vi "MW100 General Start.vi"(8 "error in (no error)":errorcluster, 11 "MW100 Input":refnum<visa-resource-name>) -> (0 "error out":errorcluster, 3 "MW100 Output":refnum<visa-resource-name>="MW100")   [LabVIEW 2016]
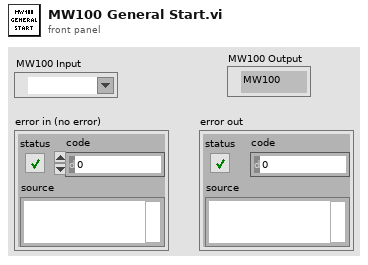
[diagram p1: front panel]
types:
  T1 = enum16{"Computation Start", "Computation stop", "Reset Computation", "Clear Computation"}
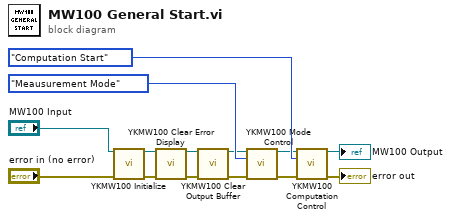
[diagram p0: block diagram]
diagram:
  n1 = call "YKMW100 Initialize.vi"("VISA session (TCPIP::)"="MW100 Input", "error in (no error)"="error in (no error)") -> ("dup VISA session"=w11:refnum<visa-resource-name>, "error out"=w8:errorcluster)  [unwired: 12 in]
  n2 = call "YKMW100 Clear Error Display.vi"("VISA session"=w11, "error in (no error)"=w8) -> ("dup VISA session"=w10:refnum<visa-resource-name>, "error out"=w9:errorcluster)  [unwired: 10 in, 2 out]
  n3 = call "YKMW100 Clear Output Buffer.vi"("VISA session"=w10, "error in (no error)"=w9) -> ("dup VISA session"=w2:refnum<visa-resource-name>, "error out"=w3:errorcluster)  [unwired: 12 in]
  n4 = call "YKMW100 Mode Control.vi"("VISA session"=w2, "Model"=enum16{"Meausurement Mode", "Setting Mode"}."Meausurement Mode", "error in (no error)"=w3) -> ("dup VISA session"=w4:refnum<visa-resource-name>, "error out"=w5:errorcluster)  [unwired: 11 in]
  n5 = call "YKMW100 Computation Control.vi"("VISA session"=w4, "Mode"=T1."Computation Start", "error in (no error)"=w5) -> ("dup VISA session"=→"MW100 Output":refnum<visa-resource-name>, "error out"=→"error out":errorcluster)  [unwired: 11 in]
